vi "Create.vi"(8 "error in (no error)":errorcluster, 10 "Command Types":T1, 11 "Command Factory in":refnum<class "Command Factory.lvclass">) -> (0 "error out":errorcluster, 2 "Command":refnum<class "Command.lvclass">, 3 "Command Factory out":refnum<class "Command Factory.lvclass">)   [LabVIEW 2015, in "Command Factory.lvclass"]
uses:
  Command Factory.lvclass
  Command/Command.lvclass
  Typedefs/Command Types.ctl
  Start Command/Start Command.lvclass
  Enable Command/Enable Command.lvclass
  Disable Command/Disable Command.lvclass
  Standby Command/Standby Command.lvclass
  Shutdown Command/Shutdown Command.lvclass
  Update Command/Update Command.lvclass
  Typedefs/FAMT Typedefs.lvlib
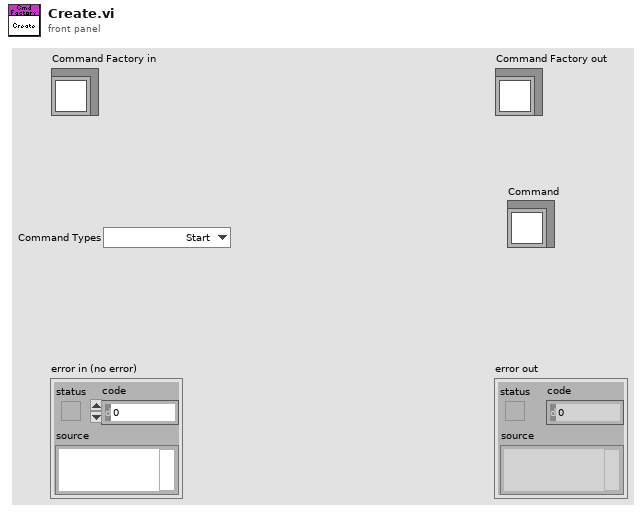
[diagram p1: front panel]
types:
  T1 = typedef "FAMT Typedefs.lvlib/Command Types.ctl" = enum16{"Start", "Enable", "Disable", "Standby", "Shutdown", "Update"}
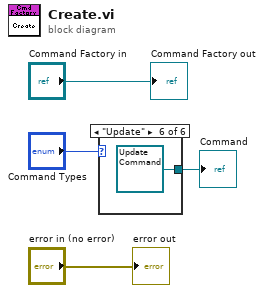
[diagram p0: block diagram]
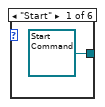
[diagram p2: hidden frame]
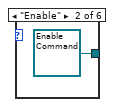
[diagram p3: hidden frame]
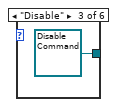
[diagram p4: hidden frame]
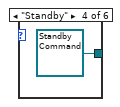
[diagram p5: hidden frame]
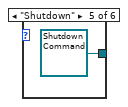
[diagram p6: hidden frame]
diagram:
  n1 = case shown="\"Update\"" "Command Types" {
    tunnel: [refnum<class "Start Command.lvclass"> refnum ("Start.lvclass") refnum<class "Enable Command.lvclass"> refnum ("Enable.lvclass") refnum<class "Disable Command.lvclass"> refnum ("Disable.lvclass") refnum<class "Standby Command.lvclass"> refnum ("Standby.lvclass") refnum<class "Shutdown Command.lvclass"> refnum ("Shutdown.lvclass") refnum<class "Update Command.lvclass"> refnum ("Update.lvclass")] -> w2
    frame "Start" {
    }
    frame "Enable" {
    }
    frame "Disable" {
    }
    frame "Standby" {
    }
    frame "Shutdown" {
    }
    frame "Update" {
    }
  }
  "Command" <- w2
  "error out" <- "error in (no error)"
  "Command Factory out" <- "Command Factory in"
